vi "listen connection LV15.vi"(8 "Bool Refnum":refnum<vi>, 10 "service name":string="192.168.1.10") -> (2 "Boolean 3":bool, 3 "data out":string)   [LabVIEW 2015]
uses:
  Galobal variable_TI.vi
panel:
  out "error out":errorcluster
  out "String":string
  out "Coordinate 3":string
  out "Numeric 2":i32
  out "error out 3":errorcluster
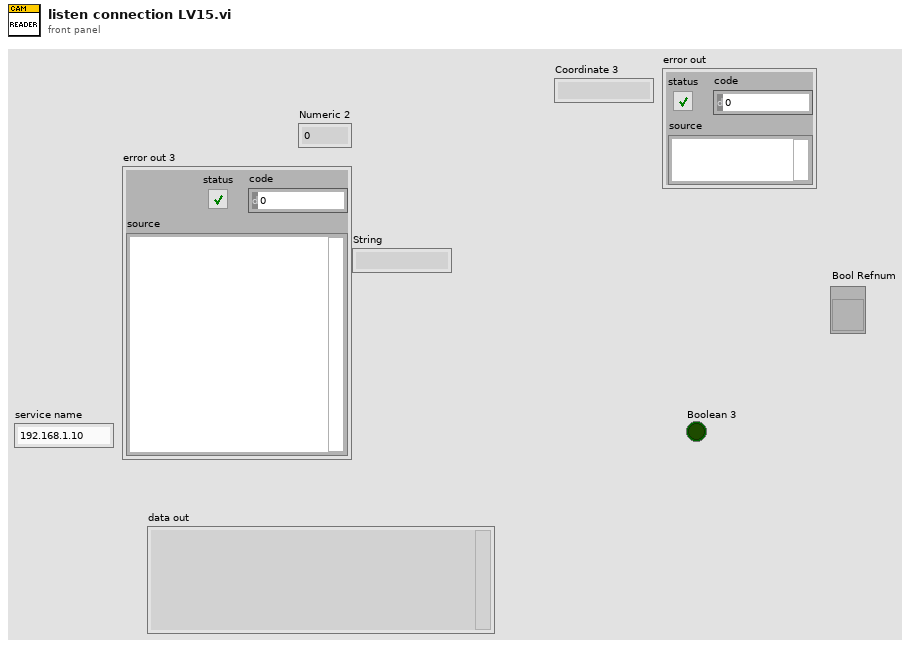
[diagram p1: front panel]
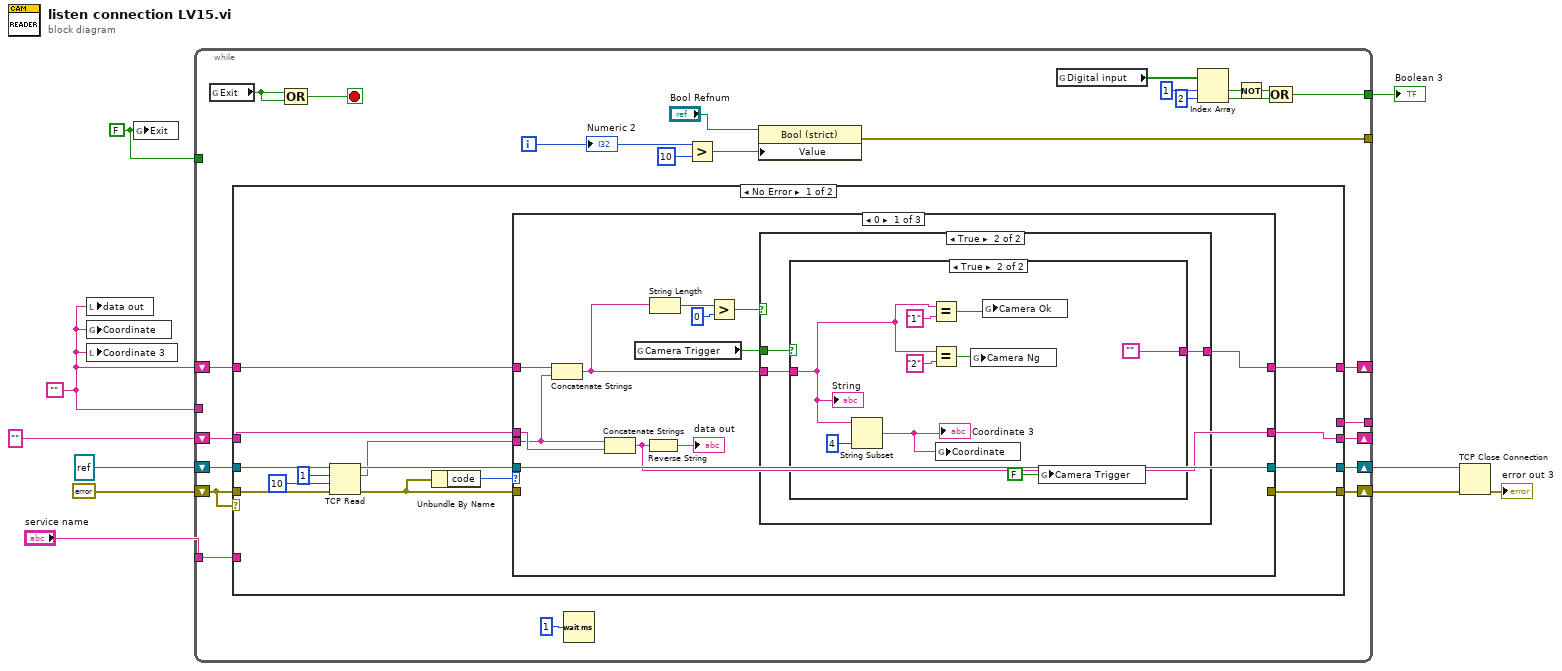
[diagram p0: block diagram]
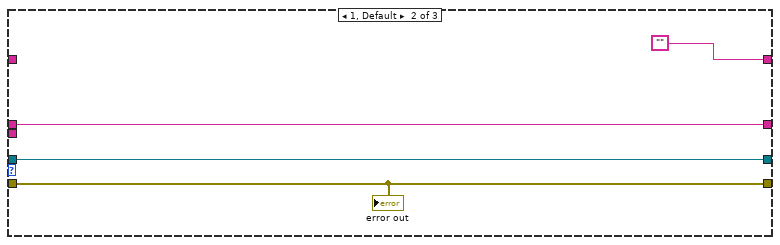
[diagram p4: hidden frame]
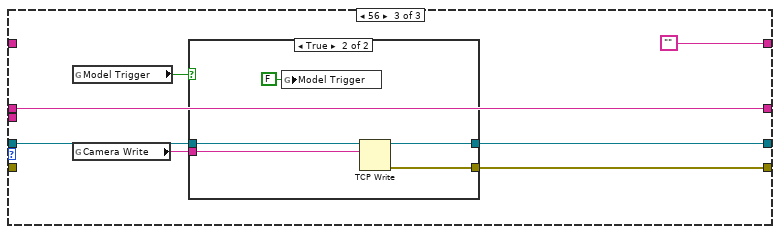
[diagram p5: hidden frame]
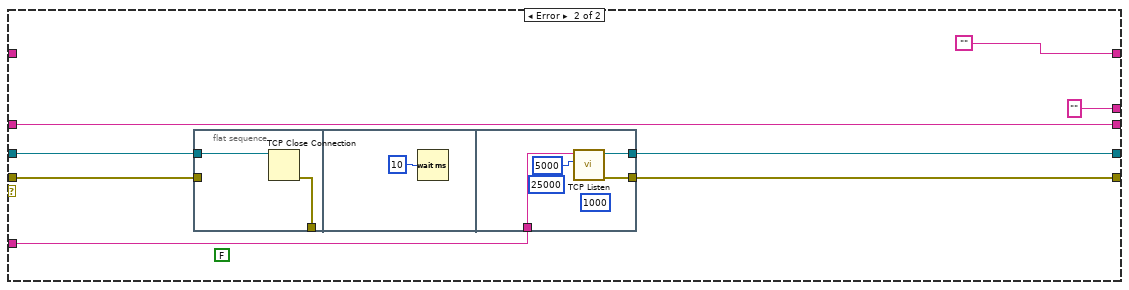
[diagram p7: hidden frame]
diagram:
  w1 = FALSE ("Exit")
  w2 = ""
  n1 = local write "data out"(w2) -> ()
  n2 = global write "Galobal variable_TI.vi" "Coordinate"(w2) -> ()
  n3 = local write "Coordinate 3"(w2) -> ()
  n4 = global write "Galobal variable_TI.vi" "Exit"(w1) -> ()
  n5 = while {
    tunnel: [w33] -> _
    shift-right: [w35] -> w10
    shift-left: refnum<k5> refnum ("connection ID") -> [w32]
    shift-right: [w34] -> w9
    shift-left: errorcluster {"status"=FALSE, "code"=0, "source"=""} ("error out") -> [w31]
    tunnel: "service name" -> [w30]
    shift-right: [w20] -> _
    shift-left: "" -> [w29]
    tunnel: [w19] -> w3
    tunnel: w2 -> [_]
    shift-right: [w16] -> _
    shift-left: w2 -> [w17]
    tunnel: [w11] -> _
    tunnel: w1 -> [_]
    i -> [w15]
    stop <- w27 stop-if-true
    n6 = global read "Galobal variable_TI.vi" "Exit"() -> (w18:bool)
    n7 = case shown="No Error" w31 {
      tunnel: [w46 w96] -> w35
      tunnel: [w45 w95] -> w34
      tunnel: [_ "" ("data out")] -> w33
      tunnel: w32 -> [w37 w100]
      tunnel: w31 -> [w36 w99]
      tunnel: w30 -> [_ w98]
      tunnel: [w40 w97] -> w20
      tunnel: w29 -> [w42 w97]
      tunnel: w17 -> [w39 _]
      tunnel: [w38 ""] -> w16
      frame No Error {
        n8 = TCP Read(connection ID=w37, bytes to read=1, error in (no error)=w36, 9:10 ("timeout ms (25000)")) -> (connection ID out=w47:refnum<k5>, data out=w43:string, error out=w44:errorcluster)  [unwired: 1 in]
        n9 = Unbundle By Name(w44) -> ("code"=w48:i32)
        n10 = case shown="0" w48 {
          tunnel: w47 -> [w61 w79 w81]
          tunnel: [w61 w79 w83] -> w46
          tunnel: [_ w76 w82] -> w45
          tunnel: w44 -> [_ w76 _]
          tunnel: w43 -> [w52 _ _]
          tunnel: [w54 w78 w86] -> w40
          tunnel: w42 -> [w55 w78 w86]
          tunnel: w39 -> [w53 _ _]
          tunnel: [w51 "" ""] -> w38
          frame 0 {
            n11 = Concatenate Strings(w53, w52) -> (w50:string)
            n12 = Concatenate Strings(w52, w55) -> (w54:string)
            n13 = global read "Galobal variable_TI.vi" "Camera Trigger"() -> (w58:bool)
            n14 = Reverse String(1:w54) -> (0:→"data out":string)
            n15 = String Length(string=w50) -> (length=w60:i32)
            n16 = Greater?(x=w60, y=0) -> (0:w59:bool)
            n17 = case shown="True" w59 {
              tunnel: w58 -> [_ w65]
              tunnel: w50 -> [w62 w64]
              tunnel: [w62 w63] -> w51
              frame False {
              }
              frame True {
                n18 = case shown="True" w65 {
                  tunnel: w64 -> [w66 w67]
                  tunnel: [w66 ""] -> w63
                  frame False {
                  }
                  frame True {
                    n19 = String Subset(string=w67, length (rest)=4 ("length (rest)")) -> (substring=w75:string)  [unwired: 1 in]
                    "Coordinate 3" <- w75
                    n20 = Equal?(x=w67, y="1") -> (x = y?=w70:bool)
                    n21 = Equal?(x=w67, y="2") -> (x = y?=w69:bool)
                    n22 = global write "Galobal variable_TI.vi" "Coordinate"(w75) -> ()
                    n23 = global write "Galobal variable_TI.vi" "Camera Ng"(w69) -> ()
                    n24 = global write "Galobal variable_TI.vi" "Camera Ok"(w70) -> ()
                    n25 = global write "Galobal variable_TI.vi" "Camera Trigger"(FALSE ("CAMERA TRIGGER")) -> ()
                    "String" <- w67
                  }
                }
              }
            }
          }
          frame 1, Default {
            "error out" <- w76
          }
          frame 56 {
            n26 = global read "Galobal variable_TI.vi" "Model Trigger"() -> (w80:bool)
            n27 = global read "Galobal variable_TI.vi" "Camera Write"() -> (w84:string)
            n28 = case shown="True" w80 {
              tunnel: w84 -> [_ w92]
              tunnel: [w87 w91] -> w83
              tunnel: [_ w90] -> w82
              tunnel: w81 -> [w87 w89]
              frame False {
              }
              frame True {
                n29 = global write "Galobal variable_TI.vi" "Model Trigger"(FALSE ("Model triger")) -> ()
                n30 = TCP Write(connection ID=w89, data in=w92) -> (connection ID out=w91:refnum<k5>, error out=w90:errorcluster)  [unwired: 2 in, 1 out]
              }
            }
          }
        }
      }
      frame Error {
        (unwired) FALSE
        n31 = flat-sequence {
          tunnel: w100 -> [w102]
          tunnel: w99 -> [_]
          tunnel: [w101] -> _
          tunnel: w98 -> [w106]
          tunnel: [w105] -> w96
          tunnel: [w104] -> w95
          frame #0 {
            n32 = TCP Close Connection(connection ID=w102) -> (error out=w101:errorcluster)  [unwired: 2 in, 1 out]
          }
          frame #1 {
            n33 = Wait (ms)(milliseconds to wait=u32 10) -> ()  [unwired: 1 out]
          }
          frame #2 {
            (unwired) 25000 ("timeout ms (wait forever: -1)")
            (unwired) 1000 ("timeout ms (wait forever: -1)")
            n34 = call <vilib>:"TCP Listen.vi"("port"=u16 5000, "service name"=w106) -> ("error out"=w104:errorcluster, "connection ID"=w105:refnum<k5>)  [unwired: 5 in, 3 out]
          }
        }
      }
    }
    n35 = Compound Arithmetic op=OR(w18, w18) -> (w27:bool)
    n36 = Wait (ms)(milliseconds to wait=u32 1) -> ()  [unwired: 1 out]
    n37 = Greater?(x=w15, y=10) -> (0:w12:bool)
    n38 = property class="Bool (strict)"(reference="Bool Refnum", "Value"=w12) -> (error out=w11:errorcluster)  [unwired: 1 in, 1 out]
    n39 = global read "Galobal variable_TI.vi" "Digital input"() -> (w26:bool[])
    n40 = Index Array(array=w26, index #1=1 ("index"), index #2=2 ("index")) -> (element #1=w23:bool, element #2=w21:bool)
    n41 = Not(x=w23) -> (.not. x?=w22:bool)
    n42 = Compound Arithmetic op=OR(w22, w21) -> (w19:bool)
    "Numeric 2" <- w15
  }
  "Boolean 3" <- w3
  n43 = TCP Close Connection(connection ID=w10, error in (no error)=w9) -> (error out=→"error out 3":errorcluster)  [unwired: 1 in, 1 out]
